vi "Power_Supply Set Reference.vi"(8 "error in (no error)":errorcluster, 10 "User Reference":i32, 11 "Power_Supply Virtual.lvclass":refnum<class "Power_Supply Virtual.lvclass">) -> (0 "error out":errorcluster)   [LabVIEW 2018, in "Power_Supply Virtual.lvclass"]
uses:
  Power_Supply Virtual.lvclass
  Power_Supply Global.vi
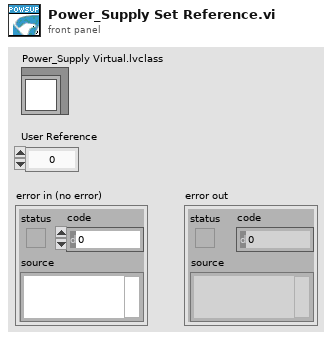
[diagram p1: front panel]
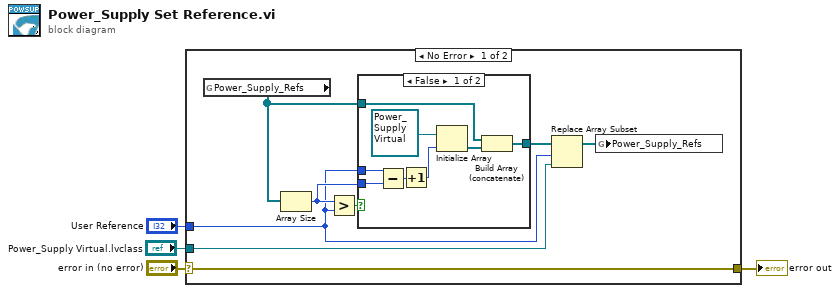
[diagram p0: block diagram]
diagram:
  n1 = case shown="No Error" "error in (no error)" {
    selector: "error in (no error)" -> [w5 w22]
    tunnel: "Power_Supply Virtual.lvclass" -> [w8 _]
    tunnel: "User Reference" -> [w6 _]
    tunnel: [w5 w22] -> w3
    frame No Error {
      n2 = global read "Power_Supply Global.vi" "Power_Supply_Refs"() -> (w9:refnum<class "Power_Supply Virtual.lvclass">[])
      n3 = Array Size(array=w9) -> (size(s)=w10:i32)
      n4 = Greater?(x=w10, y=w6) -> (0:w12:bool)
      n5 = case shown="False" w12 {
        tunnel: w6 -> [w19 _]
        tunnel: w9 -> [w20 w21]
        tunnel: w10 -> [w18 _]
        tunnel: [w15 w21] -> w11
        frame False {
          n6 = Subtract(x=w19, y=w18) -> (x-y=w17:i32)
          n7 = Increment(x=w17) -> (x+1=w16:i32)
          n8 = Initialize Array(refnum<class "Power_Supply Virtual.lvclass"> refnum ("Power_Supply Virtual.lvclass"), w16) -> (w14:refnum<class "Power_Supply Virtual.lvclass">[])
          n9 = Build Array (concatenate)(w20, w14) -> (w15:refnum<class "Power_Supply Virtual.lvclass">[])
        }
        frame True {
        }
      }
      n10 = Replace Array Subset(array=w11, new element=w8, index=w6) -> (w7:refnum<class "Power_Supply Virtual.lvclass">[])
      n11 = global write "Power_Supply Global.vi" "Power_Supply_Refs"(w7) -> ()
    }
    frame Error {
    }
  }
  "error out" <- w3
